vi "BASE_Login Screen.vi"(8 "Error In":errorcluster, 10 "Password":string, 11 "User Name":string(combo)) -> (0 "error out":errorcluster, 1 "Level":i32, 2 "Login Done":bool, 3 "User Name Out":string(combo))   [LabVIEW 2017]
uses:
  <vilib>/Utility/config.llb/Read Key (String).vi
  <vilib>/Utility/config.llb/Read Key (I32).vi
  <vilib>/Utility/config.llb/NI_LVConfig.lvlib
panel:
  in  "Cancel":bool
  in  "OK Button":bool
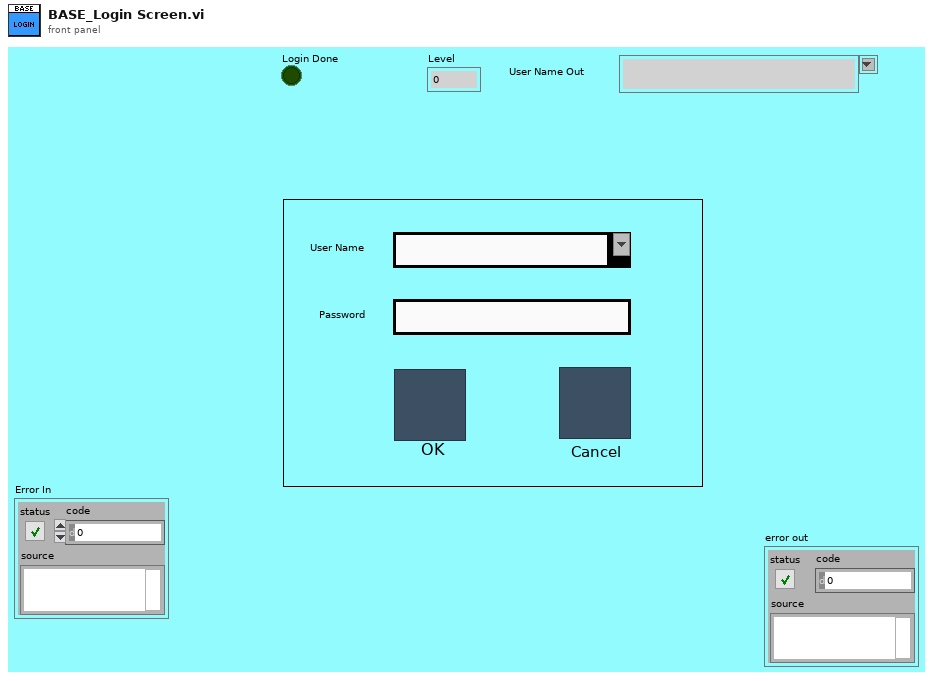
[diagram p1: front panel]
types:
  T1 = enum32{"invalid app kind", "Development System", "Run Time System", "Student Edition", "Embedded LabVIEW", "Evaluation", "Custom"}
  T2 = typedef "NI_LVConfig.lvlib/Config Data RefNum.ctl" = refnum<k1>
  T3 = enum32{"Invalid", "Standard", "Closed", "Hidden", "Minimized", "Maximized"}
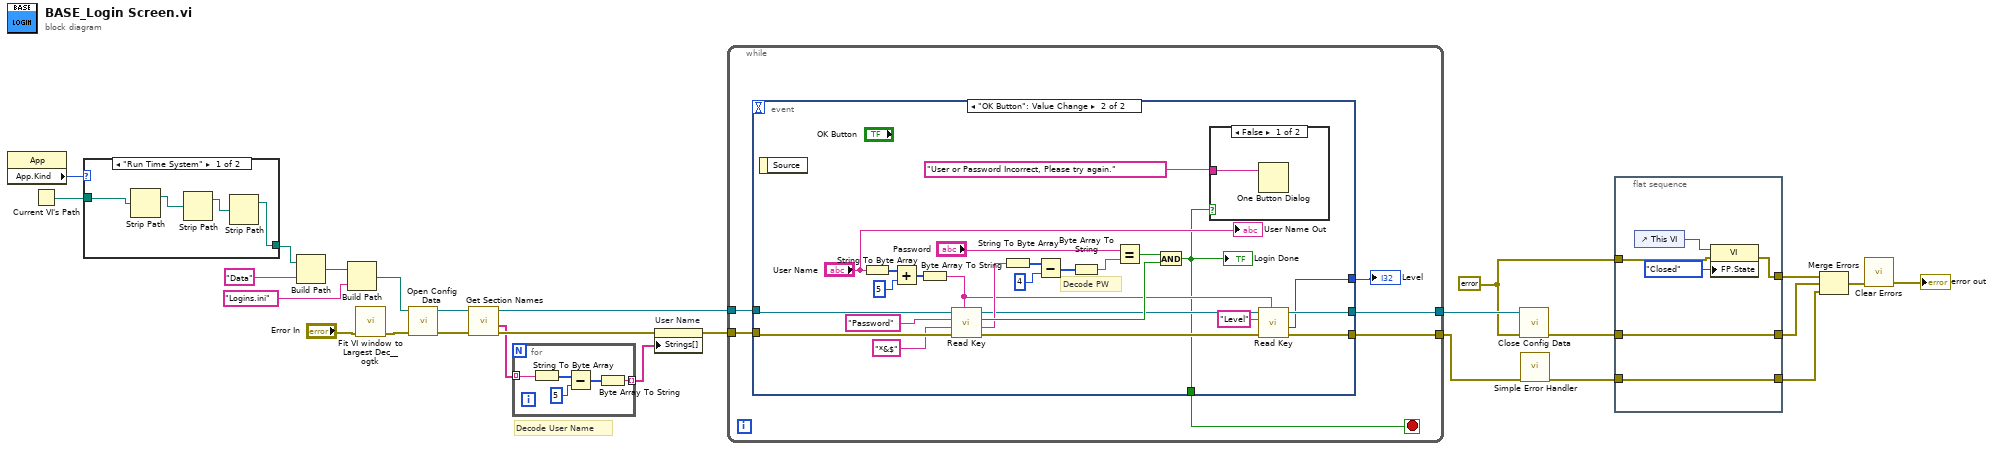
[diagram p0: block diagram]
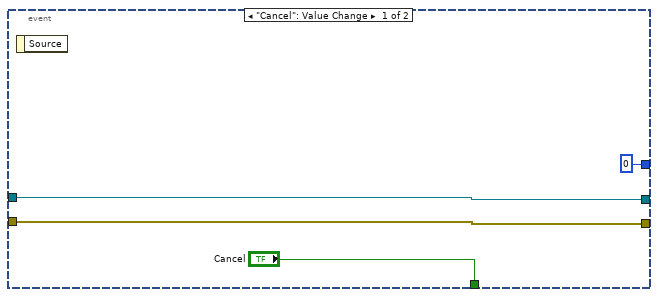
[diagram p2: hidden frame]
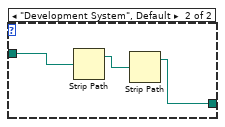
[diagram p4: hidden frame]
diagram:
  w19 = errorcluster {"status"=FALSE, "code"=0, "source"=""} ("error in (no error)")
  # "Decode User Name"
  n1 = property class="App"() -> ("App.Kind"=w26:T1)  [unwired: 2 in, 2 out]
  n2 = Current VI's Path() -> (path=w1:path)
  n3 = case shown="\"Run Time System\"" w26 {
    tunnel: w1 -> [w29 w32]
    tunnel: [w27 w31] -> w2
    frame "Run Time System" {
      n4 = Strip Path(path=w29) -> (stripped path=w30:path)  [unwired: 1 out]
      n5 = Strip Path(path=w30) -> (stripped path=w28:path)  [unwired: 1 out]
      n6 = Strip Path(path=w28) -> (stripped path=w27:path)  [unwired: 1 out]
    }
    frame "Development System", Default {
      n7 = Strip Path(path=w32) -> (stripped path=w33:path)  [unwired: 1 out]
      n8 = Strip Path(path=w33) -> (stripped path=w31:path)  [unwired: 1 out]
    }
  }
  n9 = Build Path(base path=w2, name or relative path="Data") -> (appended path=w25:path)
  n10 = Build Path(base path=w25, name or relative path="Logins.ini") -> (appended path=w24:path)
  n11 = call <userlib>:"Fit VI window to Largest Dec__ogtk.vi"("error in (no error)"="Error In") -> ("error out"=w3:errorcluster)  [unwired: 5 in, 1 out]
  n12 = call <vilib>:"Open Config Data.vi"("error in (no error)"=w3, "configuration file path"=w24) -> ("error out"=w10:errorcluster, "refnum"=w11:T2)  [unwired: 7 in, 1 out]
  n13 = call <vilib>:"Get Section Names.vi"("error in (no error)"=w10, "refnum"=w11) -> ("error out"=w8:errorcluster, "section names"=w6:string[], "refnum out"=w9:T2)  [unwired: 7 in]
  n14 = for {
    tunnel: w6 -> [w38] mode=indexing
    tunnel: [w34] -> w5 mode=indexing
    n15 = String To Byte Array(string=w38) -> (unsigned byte array=w37:u8[])
    n16 = Subtract(x=w37, y=u8 5) -> (x-y=w35:u8[])
    n17 = Byte Array To String(unsigned byte array=w35) -> (string=w34:string)
  }
  n18 = property on="User Name" class="CmbBox"(error in=w8, "Strings[]"=w5) -> (error out=w7:errorcluster)  [unwired: 1 in, 1 out]
  n19 = while {
    tunnel: [w43] -> w21
    tunnel: w9 -> [w42]
    tunnel: [w41] -> w20
    tunnel: w7 -> [w40]
    stop <- w44 stop-if-true
    n20 = event shown="[1] \"OK Button\": Value Change" {
      selector: _ -> [_ _]
      dyn-events: _ -> [_ _]
      timeout: _ -> [_ _]
      tunnel: ["Cancel" w50] -> w44
      tunnel: [w47 w54] -> w43
      tunnel: w42 -> [w47 w73]
      tunnel: [w46 w53] -> w41
      tunnel: w40 -> [w46 w72]
      tunnel: [0 ("value") w51] -> w39
      event "Cancel": Value Change {
        n21 = event-data() -> ()  [unwired: 1 in, 1 out]
      }
      event "OK Button": Value Change {
        # "Decode PW"
        n22 = event-data() -> ()  [unwired: 1 in, 1 out]
        n23 = String To Byte Array(string="User Name") -> (unsigned byte array=w61:u8[])
        n24 = Add(x=w61, y=u8 5) -> (x+y=w59:u8[])
        n25 = Byte Array To String(unsigned byte array=w59) -> (string=w57:string)
        n26 = call-poly <vilib>:"Read Key.vi"("section"=w57, "error in (no error)"=w72, "default value"="*&$", "key"="Password", "refnum"=w73) -> ("error out"=w56:errorcluster, "value"=w66:string, "found?"=w68:bool, "refnum out"=w55:T2)  [unwired: 3 in]
        n27 = String To Byte Array(string=w66) -> (unsigned byte array=w65:u8[])
        n28 = Subtract(x=w65, y=u8 4) -> (x-y=w63:u8[])
        n29 = Byte Array To String(unsigned byte array=w63) -> (string=w62:string)
        n30 = Equal?(x="Password", y=w62) -> (x = y?=w69:bool)
        n31 = And(x=w69, y=w68) -> (x .and. y?=w50:bool)
        "Login Done" <- w50
        n32 = case shown="False" w50 {
          tunnel: "User or Password Incorrect, Please try again." -> [w74 _]
          frame False {
            n33 = One Button Dialog(message=w74) -> ()  [unwired: 1 in, 1 out]
          }
          frame True {
          }
        }
        n34 = call-poly <vilib>:"Read Key.vi"("section"=w57, "error in (no error)"=w56, "key"="Level", "refnum"=w55) -> ("error out"=w53:errorcluster, "value"=w51:i32, "refnum out"=w54:T2)  [unwired: 4 in, 1 out]
        "User Name Out" <- "User Name"
      }
    }
    "Level" <- w39
  }
  n35 = call <vilib>:"Close Config Data.vi"("error in (no error)"=w19, "refnum"=w21) -> ("error out"=w14:errorcluster)  [unwired: 8 in, 1 out]
  n36 = call <vilib>:"Simple Error Handler.vi"("error in (no error)"=w20) -> ("error out"=w12:errorcluster)  [unwired: 4 in, 4 out]
  n37 = flat-sequence {
    tunnel: w19 -> [w78]
    tunnel: [w77] -> w18
    tunnel: [w76] -> w15
    tunnel: w14 -> [w76]
    tunnel: [w75] -> w13
    tunnel: w12 -> [w75]
    frame #0 {
      n38 = control-ref of="This VI"() -> (w80:refnum<vi>)
      n39 = property class="VI"(reference=w80, error in=w78, "FP.State"=T3."Closed" ("Front Panel Window:State")) -> (error out=w77:errorcluster)  [unwired: 1 out]
    }
  }
  n40 = Merge Errors(w18, w15, w13) -> (w17:errorcluster)
  n41 = call <vilib>:"Clear Errors.vi"("error in (no error)"=w17) -> ("error out"=→"error out":errorcluster)  [unwired: 5 in, 1 out]
